vi "数据存储-9229.vi"(8 "错误输入（无错误）":errorcluster, 10 "9229数据":waveform(dbl)[](array[waveform]), 11 "tdms文件输入":refnum<k34>) -> (0 "错误输出":errorcluster, 3 "tdms文件输出":refnum<k34>)   [LabVIEW 2013]
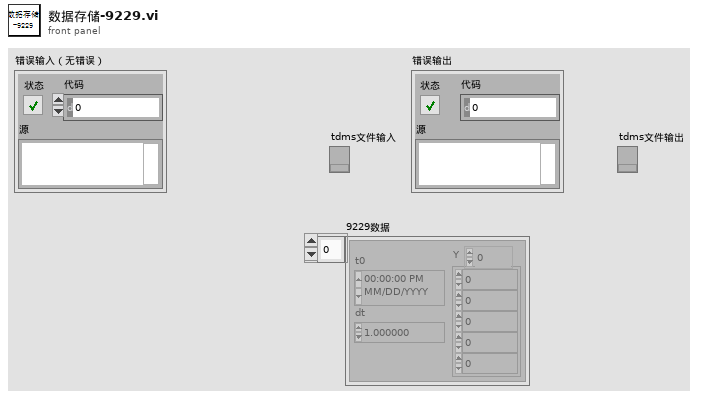
[diagram p1: front panel]
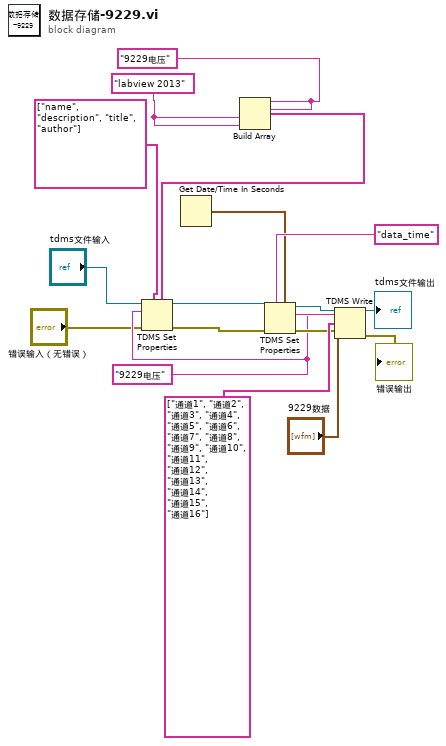
[diagram p0: block diagram]
diagram:
  w12 = "9229电压" ("组名称")
  w11 = "9229电压" ("9213")
  w7 = "labview 2013"
  n1 = Get Date/Time In Seconds() -> (seconds since 1Jan1904=w13:timestamp)
  n2 = Build Array(w11, w11, w7, w7) -> (w8:string[])
  n3 = TDMS Set Properties(5:w8, 7:string[] ["name", "description", "title", "author"] ("属性名称"), 8:"错误输入（无错误）", 10:w12, 11:"tdms文件输入") -> (0:w10:errorcluster, 3:w9:refnum<k34>)  [unwired: 1 in, 2 out]
  n4 = TDMS Set Properties(5:w13, 7:"data_time" ("属性名称"), 8:w10, 10:w12, 11:w9) -> (0:w17:errorcluster, 2:w16:string, 3:w15:refnum<k34>)  [unwired: 1 in, 1 out]
  n5 = TDMS Write(0:w15, 5:w16, 7:string[] ["通道1", "通道2", "通道3", "通道4", "通道5", "通道6", "通道7", "通道8", "通道9", "通道10", "通道11", "通道12", "通道13", "通道14", "通道15", "通道16"] ("通道名输入（无标题）"), 9:"9229数据", 11:w17) -> (4:→"tdms文件输出":refnum<k34>, 15:→"错误输出":errorcluster)  [unwired: 1 in, 2 out]
